vi "TelemetryServer_QueueStart.vi"(2 "Group":string, 3 "Telemetry":string[](array[string]), 9 "Error in (no error)":errorcluster caption="error in (no error)") -> (0 "Telemetry queues":refnum<queue>[](array[refnum]), 6 "Error out":errorcluster caption="error out", 7 "Queue references":refnum<vi>[](array[refnum]))   [LabVIEW 2009]
uses:
  TelemetryServer_Global.vi
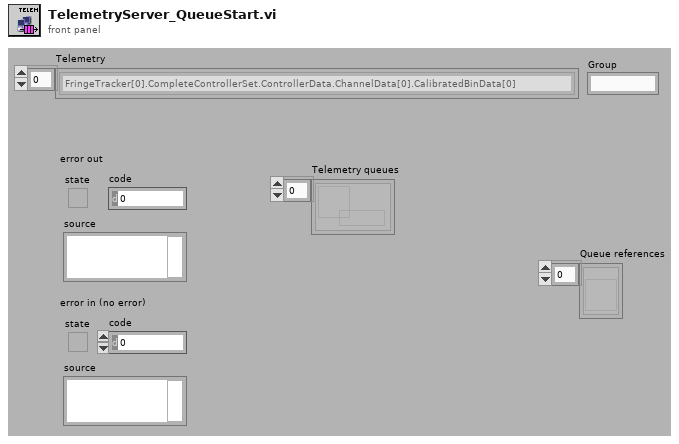
[diagram p1: front panel]
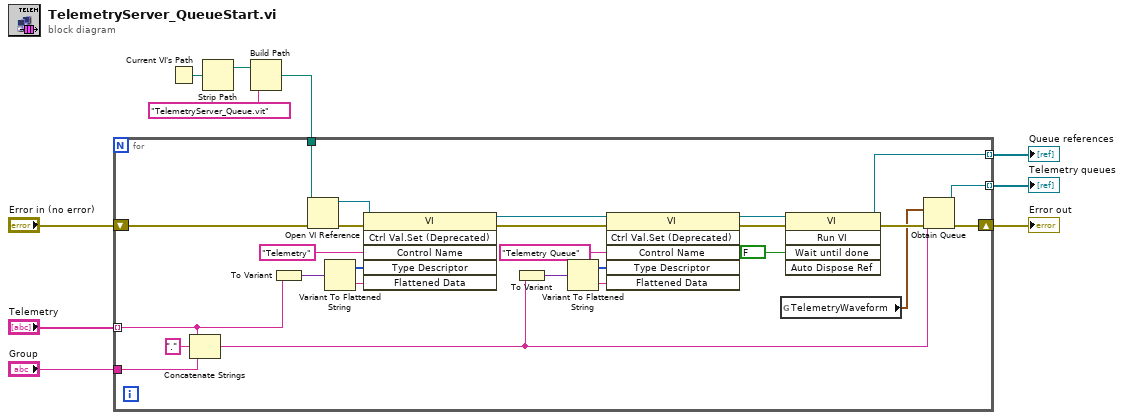
[diagram p0: block diagram]
diagram:
  n1 = Current VI's Path() -> (path=w5:path)
  n2 = Strip Path(path=w5) -> (stripped path=w6:path)  [unwired: 1 out]
  n3 = Build Path(base path=w6, name or relative path="TelemetryServer_Queue.vit" ("nom ou chemin relatif")) -> (appended path=w4:path)
  n4 = for {
    tunnel: "Telemetry" -> [w19] mode=indexing
    tunnel: "Group" -> [w18]
    tunnel: [w14] -> w1 mode=indexing
    tunnel: [w13] -> w2 mode=indexing
    tunnel: w4 -> [w11]
    shift-right: [w16] -> w8
    shift-left: "Error in (no error)" -> [w20]
    n5 = Concatenate Strings(w19, "." ("chaîne"), w18) -> (w15:string)
    n6 = To Variant(anything=w19) -> (Variant=w31:variant)
    n7 = Open VI Reference(vi path=w11, error in (no error)=w20) -> (vi reference=w34:refnum<vi>, error out=w35:errorcluster)  [unwired: 4 out]
    n8 = Variant To Flattened String(Variant=w31) -> (data string=w32:string, 1:w33:i16[])
    n9 = invoke class="VI" method="Ctrl Val.Set (Deprecated)"(reference=w34, error in=w35, "Control Name"="Telemetry" ("Nom de la commande"), "Type Descriptor"=w33, "Flattened Data"=w32) -> (reference out=w24:refnum<vi>, error out=w25:errorcluster)  [unwired: 1 in, 4 out]
    n10 = To Variant(anything=w15) -> (Variant=w28:variant)
    n11 = Variant To Flattened String(Variant=w28) -> (data string=w27:string, 1:w26:i16[])
    n12 = invoke class="VI" method="Ctrl Val.Set (Deprecated)"(reference=w24, error in=w25, "Control Name"="Telemetry Queue" ("Nom de la commande"), "Type Descriptor"=w26, "Flattened Data"=w27) -> (reference out=w22:refnum<vi>, error out=w23:errorcluster)  [unwired: 1 in, 4 out]
    n13 = global read "TelemetryServer_Global.vi" "TelemetryWaveform"() -> (w12:waveform(dbl))
    n14 = invoke class="VI" method="Run VI"(reference=w22, error in=w23, "Wait until done"=FALSE ("Attente synchrone")) -> (reference out=w13:refnum<vi>, error out=w16:errorcluster)  [unwired: 2 in, 3 out]
    n15 = Obtain Queue(name (unnamed)=w15, element data type=w12, error in (no error)=w16) -> (queue out=w14:refnum<queue>)  [unwired: 2 in, 2 out]
  }
  "Error out" <- w8
  "Queue references" <- w2
  "Telemetry queues" <- w1
